vi "SLP-cluster-to-enum.vi"(11 "Prev-Save-Load":T1) -> (3 "Prev-Save-Load enum":T2)   [LabVIEW 2016, in "SaveLoad.lvlib"]
uses:
  SaveLoad.lvlib
  controls/prev-save-load-enum.ctl
  saveloadprev.ctl
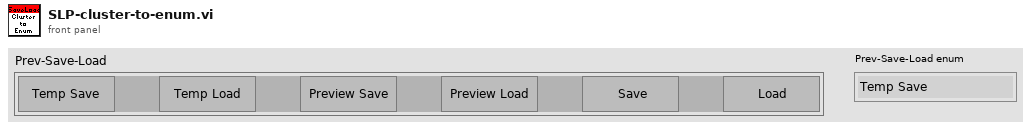
[diagram p1: front panel]
types:
  T1 = typedef "saveloadprev.ctl" = cluster{"Temp Save":bool, "Temp Load":bool, "Save":bool, "Load":bool, "Preview Save":bool, "Preview Load":bool}
  T2 = typedef "prev-save-load-enum.ctl" = enum16{"Temp Save", "Temp Load", "Save", "Load", "Preview Save", "Preview Load"}
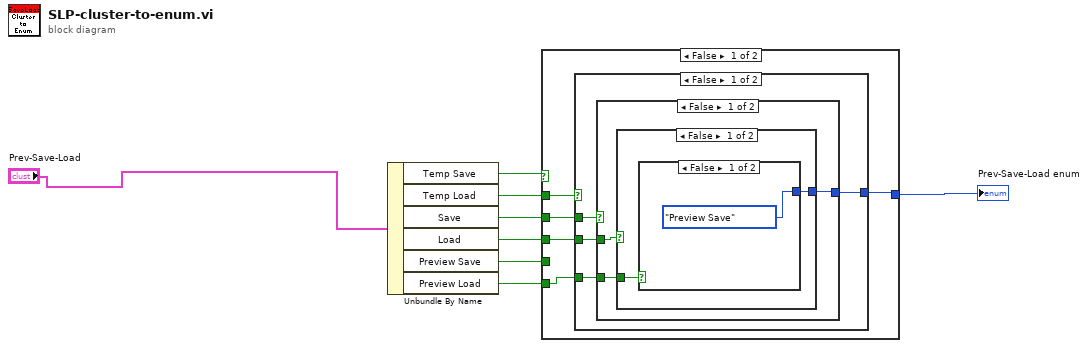
[diagram p0: block diagram]
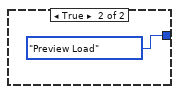
[diagram p2: hidden frame]
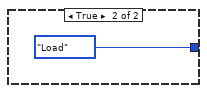
[diagram p3: hidden frame]
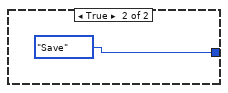
[diagram p4: hidden frame]
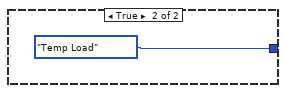
[diagram p5: hidden frame]
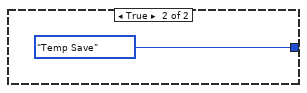
[diagram p6: hidden frame]
diagram:
  n1 = Unbundle By Name("Prev-Save-Load") -> ("Temp Save"=w2:bool, "Temp Load"=w3:bool, "Save"=w4:bool, "Load"=w5:bool, "Preview Save"=w6:bool, "Preview Load"=w7:bool)
  n2 = case shown="False" w2 {
    tunnel: [w12 prev-save-load-enum."Temp Save"] -> w8
    tunnel: w3 -> [w13 _]
    tunnel: w4 -> [w11 _]
    tunnel: w5 -> [w10 _]
    tunnel: w6 -> [_ _]
    tunnel: w7 -> [w9 _]
    frame False {
      n3 = case shown="False" w13 {
        tunnel: [w16 prev-save-load-enum."Temp Load"] -> w12
        tunnel: w11 -> [w17 _]
        tunnel: w10 -> [w15 _]
        tunnel: w9 -> [w14 _]
        frame False {
          n4 = case shown="False" w17 {
            tunnel: [w19 prev-save-load-enum."Save"] -> w16
            tunnel: w15 -> [w20 _]
            tunnel: w14 -> [w18 _]
            frame False {
              n5 = case shown="False" w20 {
                tunnel: [w22 prev-save-load-enum."Load"] -> w19
                tunnel: w18 -> [w21 _]
                frame False {
                  n6 = case shown="False" w21 {
                    tunnel: [prev-save-load-enum."Preview Save" prev-save-load-enum."Preview Load"] -> w22
                    frame False {
                    }
                    frame True {
                    }
                  }
                }
                frame True {
                }
              }
            }
            frame True {
            }
          }
        }
        frame True {
        }
      }
    }
    frame True {
    }
  }
  "Prev-Save-Load enum" <- w8
